vi "SetupSweepAndGetPeak.vi"(6 "Route Names":string[](array[string]), 7 "Cal?":bool, 8 "error in (no error)":errorcluster, 9 "Span(Hz)":dbl=26500000000.0, 10 "Center Frequency(Hz)":dbl=13250000000.0, 11 "SpecA_ESA in":refnum<class "SpecA_ESA.lvclass">) -> (0 "error out":errorcluster, 1 "FDelta(hz)":dbl, 2 "Calibrated Amplitude (dBm)":dbl, 3 "SpecA_ESA out":refnum<class "SpecA_ESA.lvclass">)   [LabVIEW 2014, in "SpecA_ESA.lvclass"]
uses:
  SpecA_ESA.lvclass
  SpecA_ESA.lvclass/SpecA_ESA.ctl
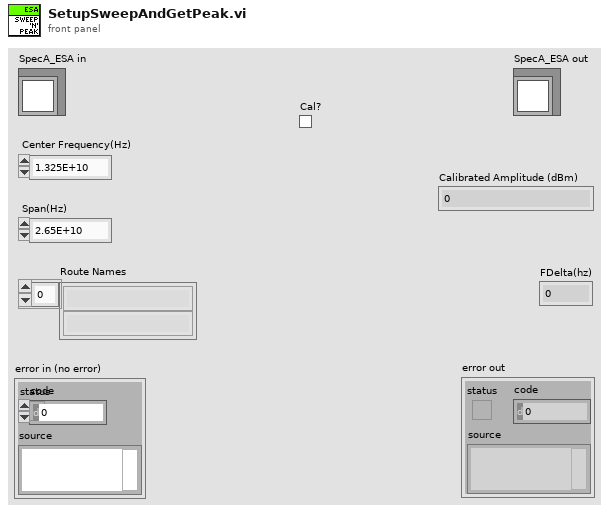
[diagram p1: front panel]
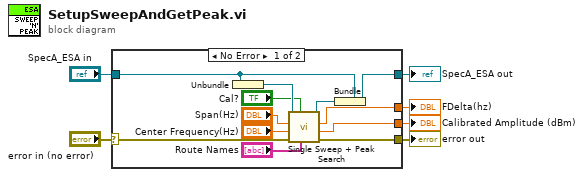
[diagram p0: block diagram]
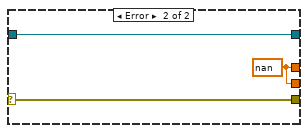
[diagram p2: hidden frame]
diagram:
  n1 = case shown="No Error" "error in (no error)" {
    selector: "error in (no error)" -> [w8 w21]
    tunnel: [w17 w21] -> w6
    tunnel: [w16 w19] -> w5
    tunnel: [w15 w19] -> w4
    tunnel: [w14 w20] -> w3
    tunnel: "SpecA_ESA in" -> [w12 w20]
    frame No Error {
      n2 = Unbundle(w12) -> (w11:refnum<visa-resource-name>)
      n3 = call "Single Sweep + Peak Search.vi"("Cal Route"="Route Names", "Cal?"="Cal?", "error in (no error)"=w8, "Center (Hz)"="Center Frequency(Hz)", "Span (Hz)"="Span(Hz)", "VISA Refnum in"=w11) -> ("error out"=w17:errorcluster, "Calibrated Marker Amplitude"=w16:dbl, "Marker Position"=w15:dbl, "VISA Refnum out"=w13:refnum<visa-resource-name>)  [unwired: 2 in]
      n4 = Bundle(cluster=w12, w13) -> (w14:refnum<class "SpecA_ESA.lvclass">)
    }
    frame Error {
      w19 = nan ("Marker Position")
    }
  }
  "error out" <- w6
  "SpecA_ESA out" <- w3
  "FDelta(hz)" <- w4
  "Calibrated Amplitude (dBm)" <- w5
